vi "Read Gyro Rio.vi"(0 "Reinit":bool) -> (1 "integral x(t)":dbl format="%0.2f", 2 "integral y(t)":dbl format="%0.2f", 3 "integral z(t)":dbl format="%0.2f")   [LabVIEW 2015]
uses:
  <vilib>/myRIO/Instrument Drivers/Onboard IO/I2C/typedefs/I2C User Configuration.ctl
  <vilib>/myRIO/Instrument Drivers/Onboard IO/I2C/typedefs/I2C Transfer Rate.ctl
  <vilib>/myRIO/Instrument Drivers/Onboard IO/I2C/typedefs/I2C Reference.ctl
  <vilib>/myRIO/Common/Instrument Driver Framework/Utilities/typedefs/myRIO Generic Hardware Reference.ctl
  <vilib>/myRIO/Common/Instrument Driver Framework/Utilities/typedefs/Hardware Version Enum.ctl
  <vilib>/myRIO/Common/Instrument Driver Framework/Utilities/typedefs/myRIO v1.0 Reference.ctl
  <vilib>/myRIO/Common/Instrument Driver Framework/Utilities/typedefs/Generic FPGA Reference.ctl
  <vilib>/myRIO/Common/Instrument Driver Framework/myRIO v1.0/I2C/typedefs/I2C Channels Enum.ctl
  <vilib>/myRIO/Instrument Drivers/Onboard IO/I2C/typedefs/I2C Configuration.ctl
  <vilib>/userdefined/High Color/nirio_resource_hc.ctl
  <vilib>/myRIO/Common/Instrument Driver Framework/myRIO v1.0/I2C/vis/myRIO v1.1 Open I2C.vi
  <vilib>/myRIO/Common/Instrument Driver Framework/Utilities/vis/Validate Channels.vi
  <vilib>/myRIO/Common/Instrument Driver Framework/myRIO v1.0/I2C/vis/myRIO v1.0 Reserve I2C.vi
  <vilib>/myRIO/Common/Instrument Driver Framework/myRIO v1.0/I2C/vis/myRIO v1.0 Close I2C.vi
  <vilib>/myRIO/Common/Instrument Driver Framework/myRIO v1.0/I2C/vis/myRIO v1.0 Build MUX Configuration I2C.vi
  <vilib>/myRIO/Common/Instrument Driver Framework/myRIO v1.0/Resource Manager/vis/myRIO v1.0 Reserve Channel List.vi
  <vilib>/myRIO/Common/Instrument Driver Framework/myRIO v1.0/I2C/vis/myRIO v1.0 Unreserve I2C.vi
  <vilib>/myRIO/Common/Instrument Driver Framework/myRIO v1.0/Resource Manager/vis/myRIO v1.0 Create Configuration List.vi
  <vilib>/myRIO/Common/Instrument Driver Framework/myRIO v1.0/Resource Manager/vis/myRIO v1.0 Reserve Channel.vi
  <vilib>/myRIO/Common/Instrument Driver Framework/myRIO v1.0/Resource Manager/vis/myRIO v1.0 Unreserve Channel.vi
  <vilib>/myRIO/Common/Instrument Driver Framework/myRIO v1.0/Resource Manager/vis/myRIO v1.0 Unreserve Channel List.vi
  <vilib>/myRIO/Common/Instrument Driver Framework/myRIO v1.0/Resource Manager/vis/myRIO v1.0 Build Mutex Name.vi
  <vilib>/Utility/VariantDataType/GetNumericInfo.vi
  <vilib>/Utility/error.llb/Error Cluster From Error Code.vi
  <vilib>/myRIO/Common/Instrument Driver Framework/myRIO v1.0/myRIO v1.1 Open.vi
  <vilib>/myRIO/Common/Instrument Driver Framework/Utilities/vis/IO Manager.vi
  <vilib>/myRIO/Common/Instrument Driver Framework/Utilities/vis/Configuration Manager.vi
  <vilib>/myRIO/Common/Instrument Driver Framework/myRIO v1.0/Resource Manager/vis/myRIO v1.0 Configure IO.vi
  <vilib>/myRIO/Common/Instrument Driver Framework/myRIO v1.0/myRIO v1.0 Close.vi
  <vilib>/myRIO/Common/Instrument Driver Framework/myRIO v1.0/I2C/vis/myRIO v1.0 Configure I2C.vi
  <vilib>/myRIO/Common/Instrument Driver Framework/myRIO v1.0/I2C/vis/myRIO v1.0 Write I2C.vi
  <vilib>/myRIO/Common/Instrument Driver Framework/myRIO v1.0/I2C/vis/myRIO v1.0 Read I2C.vi
  <vilib>/myRIO/Common/Instrument Driver Framework/myRIO v1.0/I2C/vis/myRIO v1.0 Shutdown I2C.vi
  <vilib>/myRIO/Instrument Drivers/Onboard IO/I2C/vis/myRIO I2C Open.xnode
  <vilib>/myRIO/Instrument Drivers/Onboard IO/I2C/I2C.lvlib
  <vilib>/ptbypt/NI_PtbyPt.lvlib
panel:
  out "z":i16
  out "x":i16
  out "y":i16
  out "Bytes Read":u8[](array[numeric]) format="%b"
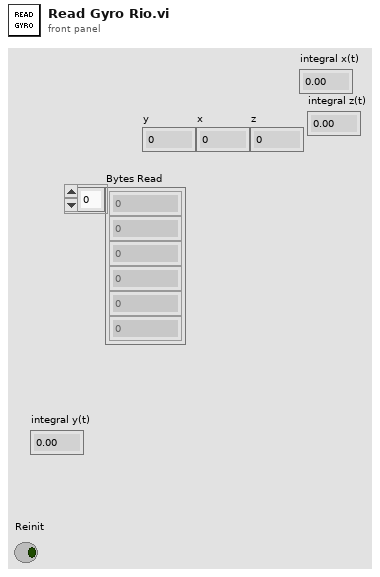
[diagram p1: front panel]
types:
  T1 = typedef "I2C.lvlib/I2C User Configuration.ctl" = cluster{"I2C Transfer Rate":T2}
  T2 = typedef "I2C.lvlib/I2C Transfer Rate.ctl" = enum16{"Standard mode (100 kbps)", "Fast mode (400 kbps)"}
  T3 = typedef "nirio_resource_hc.ctl" = tag
  T4 = typedef "Hardware Version Enum.ctl" = enum16{"Unknown", "myRIO-1900", "myRIO-1950", "roboRIO"}
  T5 = typedef "I2C.lvlib/I2C Reference.ctl" = cluster{"myRIO Reference":T6, "I2C Channels Enum":T9, "I2C Configuration":T10}
  T6 = typedef "myRIO Generic Hardware Reference.ctl" = cluster{"myRIO Model":T4, "myRIO Hardware Reference":T7}
  T7 = typedef "myRIO v1.0 Reference.ctl" = cluster{"Generic FPGA Reference":T8, "Allow multiple opens":bool}
  T8 = typedef "Generic FPGA Reference.ctl" = refnum<k20>
  T9 = typedef "I2C Channels Enum.ctl" = enum16{"Not Connected", "A/I2C", "B/I2C", "I2C/I2C"}
  T10 = typedef "I2C.lvlib/I2C Configuration.ctl" = cluster{"I2C Transfer Rate":T2}
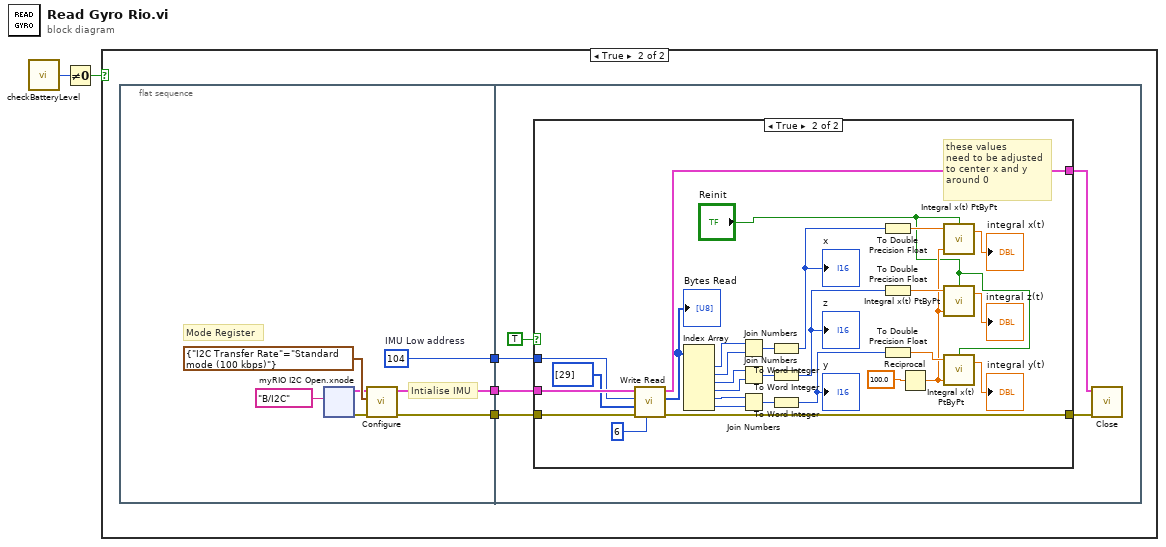
[diagram p0: block diagram]
diagram:
  n1 = call "checkBatteryLevel.vi"() -> ("Battery State"=w2:i32)
  n2 = Not Equal To 0?(x=w2) -> (x != 0?=w1:bool)
  n3 = case shown="True" w1 {
    frame False {
    }
    frame True {
      n4 = flat-sequence {
        tunnel: [w7] -> w5
        tunnel: [w8] -> w4
        tunnel: [w6] -> w3
        tunnel: w5 -> [w34]
        tunnel: w4 -> [w33]
        tunnel: w3 -> [w32]
        frame #0 {
          w8 = u8 104  # IMU Low address
          # "Mode Register"
          # "Intialise IMU"
          n5 = xnode "myRIO I2C Open.xnode"("Channel Name"=tag "B/I2C") -> ("error out"=w12:errorcluster, "I2C Ref Out"=w10:T5)  [unwired: 2 in]
          n6 = call <vilib>:"Configure.vi"("error in (no error)"=w12, "I2C User Configuration"=T1 {"I2C Transfer Rate"=enum."Standard mode (100 kbps)"}, "I2C Ref In"=w10) -> ("error out"=w6:errorcluster, "I2C Ref Out"=w7:T5)  [unwired: 7 in]
        }
        frame #1 {
          n7 = case shown="True" TRUE {
            tunnel: w34 -> [w35 w65]
            tunnel: w33 -> [_ w64]
            tunnel: w32 -> [w36 w40]
            tunnel: [w35 w39] -> w30
            tunnel: [w36 w38] -> w29
            frame False {
            }
            frame True {
              # "these values\nneed to be adjusted\nto center x and y\naround 0"
              n8 = call <vilib>:"Write Read.vi"("Byte Count"=u32 6, "error in (no error)"=w40, "Bytes to Write"=u8[] [29], "Slave Address (7-bit)"=w64, "I2C Ref In"=w65) -> ("error out"=w38:errorcluster, "Bytes Read"=w56:u8[], "I2C Ref Out"=w39:T5)  [unwired: 3 in]
              "Bytes Read" <- w56
              n9 = Index Array(array=w56) -> (element #1=w59:u8, element #2=w58:u8, element #3=w53:u8, element #4=w52:u8, element #5=w55:u8, element #6=w54:u8)  [unwired: 6 in]
              n10 = Join Numbers(hi=w59, lo=w58) -> ((hi.lo)=w57:u16)
              n11 = Join Numbers(hi=w53, lo=w52) -> ((hi.lo)=w60:u16)
              n12 = Join Numbers(hi=w55, lo=w54) -> ((hi.lo)=w61:u16)
              n13 = To Word Integer(number=w57) -> (16bit integer=w51:i16)
              "x" <- w51
              n14 = To Word Integer(number=w60) -> (16bit integer=w46:i16)
              "z" <- w46
              n15 = To Word Integer(number=w61) -> (16bit integer=w47:i16)
              "y" <- w47
              n16 = To Double Precision Float(number=w51) -> (double precision float=w50:dbl)
              n17 = To Double Precision Float(number=w46) -> (double precision float=w45:dbl)
              n18 = To Double Precision Float(number=w47) -> (double precision float=w48:dbl)
              n19 = Reciprocal(x=100.0) -> (1/x=w44:dbl)
              n20 = call <vilib>:"Integral x(t) PtByPt.vi"("initialize"="Reinit", "dt"=w44, "x"=w50) -> ("integral x(t)"=→"integral x(t)":dbl)  [unwired: 1 in, 1 out]
              n21 = call <vilib>:"Integral x(t) PtByPt.vi"("initialize"="Reinit", "dt"=w44, "x"=w45) -> ("integral x(t)"=→"integral z(t)":dbl)  [unwired: 1 in, 1 out]
              n22 = call <vilib>:"Integral x(t) PtByPt.vi"("initialize"="Reinit", "dt"=w44, "x"=w48) -> ("integral x(t)"=→"integral y(t)":dbl)  [unwired: 1 in, 1 out]
            }
          }
          n23 = call <vilib>:"Close.vi"("error in (no error)"=w29, "I2C Ref In"=w30) -> ()  [unwired: 9 in, 1 out]
        }
      }
    }
  }
